vi "FindDisplayStringForTag.vi"(8 "error in (no error)":errorcluster, 10 "Tag":string, 11 "Tree Refnum":refnum<vi>) -> (0 "error out":errorcluster, 1 "Disabled":string, 2 "Display String":string, 3 "Tree Refnum out":refnum<vi>)   [LabVIEW 2017, in "TreeSerializer.lvlib"]
uses:
  TreeSerializer.lvlib
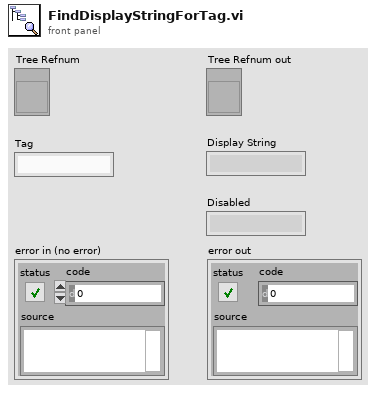
[diagram p1: front panel]
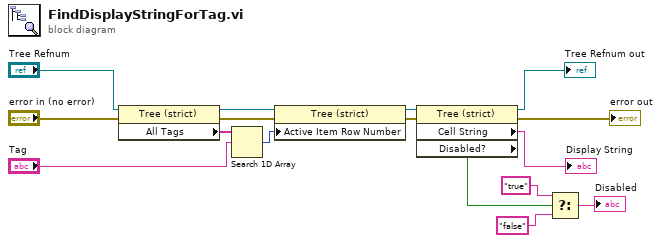
[diagram p0: block diagram]
diagram:
  n1 = property class="Tree (strict)"(reference="Tree Refnum", error in="error in (no error)") -> (reference out=w11:refnum<vi>, error out=w5:errorcluster, "All Tags"=w15:string[])
  n2 = Search 1D Array(1D array=w15, element="Tag") -> (index of element=w13:i32)  [unwired: 1 in]
  n3 = property class="Tree (strict)"(reference=w11, error in=w5, "Active Item Row Number"=w13) -> (reference out=w12:refnum<vi>, error out=w6:errorcluster)
  n4 = property class="Tree (strict)"(reference=w12, error in=w6) -> (reference out=→"Tree Refnum out":refnum<vi>, error out=→"error out":errorcluster, "Cell String"=→"Display String":string, "Disabled?"=w4:bool)
  n5 = Select(t="true" ("Active Cell:String"), s=w4, f="false" ("Active Cell:String")) -> (s? t:f=→"Disabled":string)
